vi "Add Copyright.vi"(8 "error in (no error)":errorcluster, 9 "Copyright Text":string, 10 "VI Index":i32, 11 "VI Data":T1[](array[typedef])) -> (0 "error out":errorcluster, 3 "VI Data out":T1[](array[typedef]))   [LabVIEW 2023, in "VI Properties Editor.lvlib"]
uses:
  VI Properties Editor.lvlib
  CTLs/VI Data.ctl
  <vilib>/picture/picture.llb/imagedata.ctl
  CTLs/VI Properties.ctl
  CTLs/Control Properties.ctl
  <vilib>/Utility/error.llb/Trim Whitespace One-Sided.vi
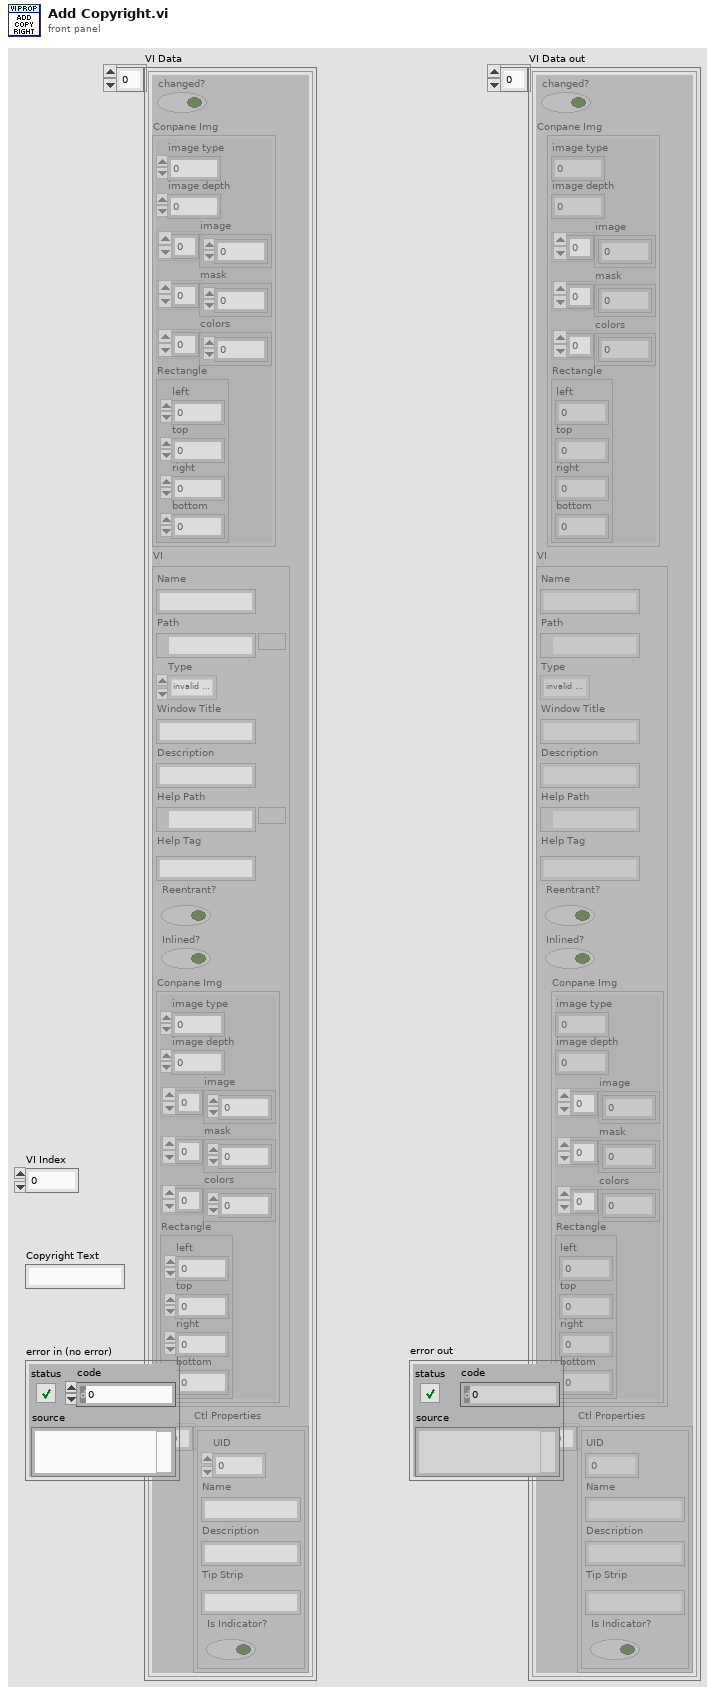
[diagram p1: front panel]
types:
  T1 = typedef "VI Properties Editor.lvlib/VI Data.ctl" = cluster{"changed?":bool, "Conpane Img":T2, "VI":T3, "Ctl Properties":T4[]}
  T2 = typedef "imagedata.ctl" = cluster{"image type":i32, "image depth":i32, "image":u8[], "mask":u8[], "colors":u32[], "Rectangle":cluster{"left":i16, "top":i16, "right":i16, "bottom":i16}}
  T3 = typedef "VI Properties Editor.lvlib/VI Properties.ctl" = cluster{"Name":string, "Path":path, "Type":enum32{"invalid VI type", "Standard VI", "Control VI", "Global VI", "Polymorphic VI", "Configuration VI", "SubSystem", "Facade VI", "Method VI", "Statechart Diagram VI"}, "Window Title":string, "Description":string, "Help Path":path, "Help Tag":string, "Reentrant?":bool, "Inlined?":bool, "Conpane Img":T2}
  T4 = typedef "VI Properties Editor.lvlib/Control Properties.ctl" = cluster{"UID":i32, "Name":string, "Description":string, "Tip Strip":string, "Is Indicator?":bool}
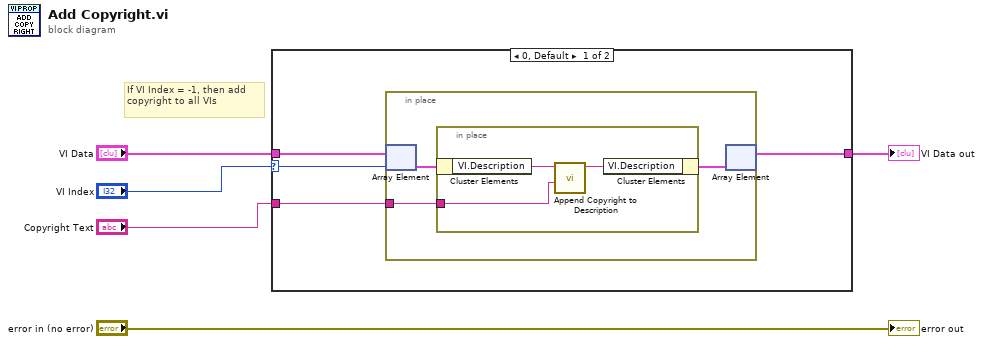
[diagram p0: block diagram]
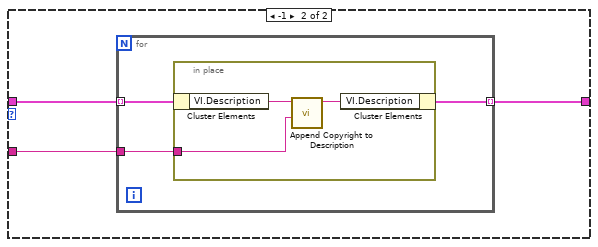
[diagram p2: hidden frame]
diagram:
  # "If VI Index = -1, then add copyright to all VIs"
  n1 = case shown="0, Default" "VI Index" {
    selector: "VI Index" -> [w8 _]
    tunnel: "VI Data" -> [w9 w18]
    tunnel: "Copyright Text" -> [w7 w17]
    tunnel: [w6 w16] -> w1
    frame 0, Default {
      n2 = in-place {
        in-place-border: w7 -> [w10]
        n3 = in-place-array #1(w9, w8) -> (w12:T1)
        n4 = in-place {
          in-place-border: w10 -> [w14]
          n5 = in-place-cluster #2(w12) -> ("VI.Description"=w15:string)
          n6 = call "Append Copyright to Description.vi"("Copyright"=w14, "Description in"=w15) -> ("Description out"=w13:string)  [unwired: 9 in]
          n7 = in-place-cluster #2("VI.Description"=w13) -> (w11:T1)
        }
        n8 = in-place-array #1(w11) -> (w6:T1[])  [unwired: 1 out]
      }
    }
    frame -1 {
      n9 = for {
        tunnel: w18 -> [w21] mode=indexing
        tunnel: w17 -> [w20]
        tunnel: [w19] -> w16 mode=indexing
        n10 = in-place {
          in-place-border: w20 -> [w23]
          n11 = in-place-cluster #3(w21) -> ("VI.Description"=w24:string)
          n12 = call "Append Copyright to Description.vi"("Copyright"=w23, "Description in"=w24) -> ("Description out"=w22:string)  [unwired: 9 in]
          n13 = in-place-cluster #3("VI.Description"=w22) -> (w19:T1)
        }
      }
    }
  }
  "VI Data out" <- w1
  "error out" <- "error in (no error)"
